vi "UTIL_Initialize Queue v1_0_0.vi"(5 "index of Single\nQueue to Use":i32, 6 "Token":string[](array[string])=["?"], 7 "Use Queue Array?":bool=TRUE, 8 "error in":errorcluster, 9 "Manual Queue Array In":string[](array[string]), 10 "Manual Enqueue":bool=TRUE, 11 "Path":path) -> (0 "error out":errorcluster, 1 "Queue Array":string[](array[string]), 2 "Token String":string, 3 "queue out":refnum<queue>)   [LabVIEW 2009]
doc: "UTIL_Initialize Queue v1_0_0.vi\n\nRetrirves info from the queue so that you can pre-load the state machine.\n\nAllows that information to be placed on the queue or used for other purposes.\n\nCreated 2006 by\nJ. Daren Suntych\nNational Analytics\n970-397-0764"
panel:
  in  "timeout in ms (10)":i32=100
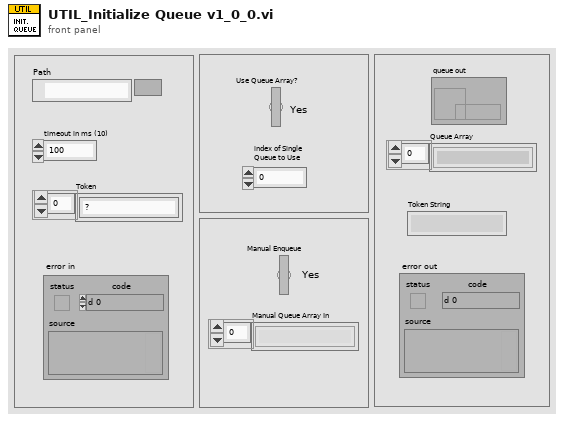
[diagram p1: front panel]
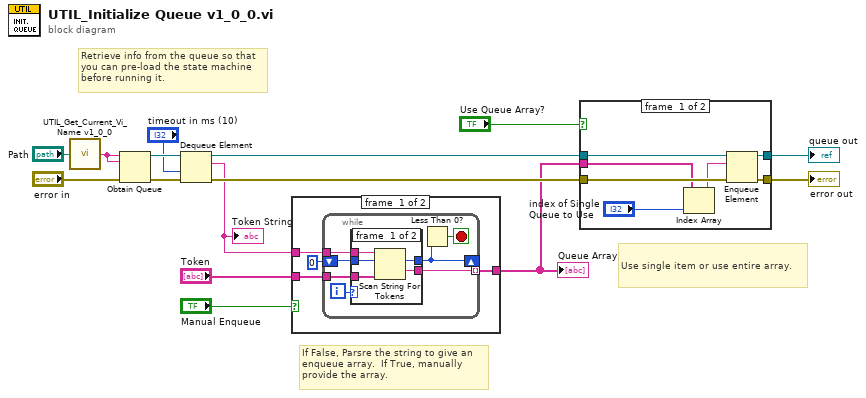
[diagram p0: block diagram]
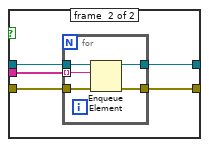
[diagram p2: hidden frame]
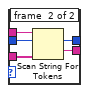
[diagram p3: hidden frame]
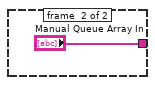
[diagram p4: hidden frame]
diagram:
  # "Use single item or use entire array."
  # "If False, Parsre the string to give an enqueue array.  If True, manually provide the array."
  # "Retrieve info from the queue so that you can pre-load the state machine before running it."
  n1 = call "UTIL_Get_Current_Vi_Name v1_0_0.vi"("Path"="Path") -> ("Name Minus Extention"=w2:string)  [unwired: 14 out]
  n2 = Obtain Queue(name (unnamed)=w2, element data type=w2, error in (no error)="error in") -> (queue out=w15:refnum<queue>, error out=w14:errorcluster)  [unwired: 2 in, 1 out]
  n3 = Dequeue Element(queue=w15, timeout in ms (-1)="timeout in ms (10)", error in (no error)=w14) -> (queue out=w10:refnum<queue>, element=w9:string, error out=w11:errorcluster)  [unwired: 1 out]
  "Token String" <- w9
  n4 = case shown="False" "Manual Enqueue" {
    tunnel: "Token" -> [w19 _]
    tunnel: w9 -> [w18 _]
    tunnel: [w16 "Manual Queue Array In"] -> w8
    frame #0 {
      n5 = while {
        tunnel: w19 -> [w26]
        tunnel: w18 -> [w25]
        shift-right: [w21] -> _
        shift-left: 0 ("offset past token") -> [w23]
        tunnel: [w20] -> w16 mode=indexing
        i -> [w24]
        stop <- w22 stop-if-true
        n6 = case shown="..0" w24 {
          tunnel: w26 -> [w30 w35]
          tunnel: w25 -> [w31 w36]
          tunnel: w23 -> [w29 w34]
          tunnel: [w28 w33] -> w21
          tunnel: [w27 w32] -> w20
          frame #0 {
            n7 = Scan String For Tokens(6:w30, 8:w29, 9:w31) -> (1:w27:string, 2:w28:i32)  [unwired: 5 out]
          }
          frame #1 {
            n8 = Scan String For Tokens(6:w35, 8:w34, 9:w36) -> (1:w32:string, 2:w33:i32)  [unwired: 5 out]
          }
        }
        n9 = Less Than 0?(x=w21) -> (x < 0?=w22:bool)
      }
    }
    frame #1 {
    }
  }
  "Queue Array" <- w8
  n10 = case shown="True" "Use Queue Array?" {
    tunnel: w11 -> [w41 w49]
    tunnel: w10 -> [w44 w48]
    tunnel: w8 -> [w40 w47]
    tunnel: [w43 w46] -> w7
    tunnel: [w42 w45] -> w6
    frame #0 {
      n11 = Index Array(array=w40, index="index of Single\nQueue to Use") -> (element=w39:string)
      n12 = Enqueue Element(queue=w44, element=w39, error in (no error)=w41) -> (queue out=w43:refnum<queue>, error out=w42:errorcluster)  [unwired: 2 out]
    }
    frame #1 {
      n13 = for {
        tunnel: w49 -> [w54]
        tunnel: w48 -> [w53]
        tunnel: w47 -> [w52] mode=indexing
        tunnel: [w51] -> w46
        tunnel: [w50] -> w45
        n14 = Enqueue Element(queue=w53, element=w52, error in (no error)=w54) -> (queue out=w51:refnum<queue>, error out=w50:errorcluster)  [unwired: 2 out]
      }
    }
  }
  "queue out" <- w7
  "error out" <- w6
